vi "Decode String Array.vi"(11 "Encoded String":string) -> (3 "Strings":string[](array[string]))   [LabVIEW 2017]
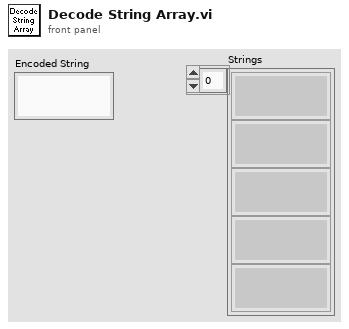
[diagram p1: front panel]
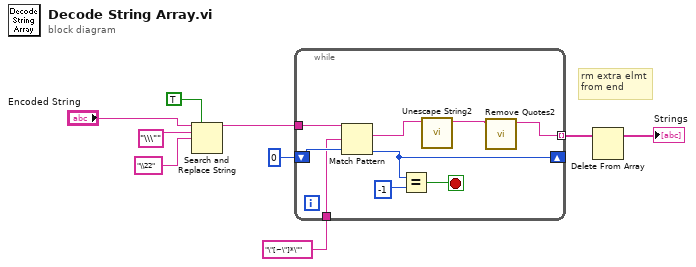
[diagram p0: block diagram]
diagram:
  # "rm extra elmt\nfrom end"
  n1 = Search and Replace String(replace all?=TRUE ("replace all? (F)"), input string="Encoded String", search string="\\\"" ("regular expression"), replace string="\\22" ("regular expression")) -> (result string=w5:string)  [unwired: 4 in, 3 out]
  n2 = while {
    tunnel: w5 -> [w13]
    shift-right: [w17] -> _
    shift-left: 0 -> [w18]
    tunnel: [w10] -> w2 mode=indexing
    tunnel: "\"[~\"]*\"" ("regular expression") -> [w14]
    stop <- w15 stop-if-true
    n3 = Match Pattern(string=w13, regular expression=w14, offset (0)=w18) -> (match substring=w12:string, offset past match=w17:i32)  [unwired: 2 out]
    n4 = Equal?(x=w17, y=-1) -> (x = y?=w15:bool)
    n5 = call <vilib>:"Unescape String2.vi"("string"=w12) -> ("parsed string"=w11:string)  [unwired: 10 in]
    n6 = call <vilib>:"Remove Quotes2.vi"("string"=w11) -> ("without quotes"=w10:string)  [unwired: 8 in, 2 out]
  }
  n7 = Delete From Array(array=w2) -> (array with subset deleted=→"Strings":string[])  [unwired: 2 in, 1 out]
